vi "BATCH 4.vi"() -> ()   [LabVIEW 2019]
uses:
  <vilib>/LabVIEW Interface for Arduino/Type Defs/Pin Mode.ctl
  <vilib>/LabVIEW Interface for Arduino/LabVIEW Interface for Arduino.lvlib
  <vilib>/ptbypt/NI_PtbyPt.lvlib
panel:
  out "Boolean 7":bool
  out "Boolean 6":bool
  out "Boolean 5":bool
  out "Boolean 4":bool
  out "Boolean 2":bool
  out "Boolean":bool
  in  "stop":bool
  out "String":string="Device under standby/Monitoring Mode"
  out "O2 Valve ON/OFF Status":bool
  out "Respiration Graph":dynamicdata(graph)
  out "Sensor Output Voltage":dbl(knob) scale=0.0..5.0
  # "O2 INHALE LIMITER"
  # "TEAM MEMBERS' NAMES:\n\nJANANISHREE V (191BM119)\nKAVINKUMAR V S (191BM121)\nKAVIYASRI S (191BM122)\nKISHORE S (191BM123)\nNAVYA C PRAKASH (191BM128)"
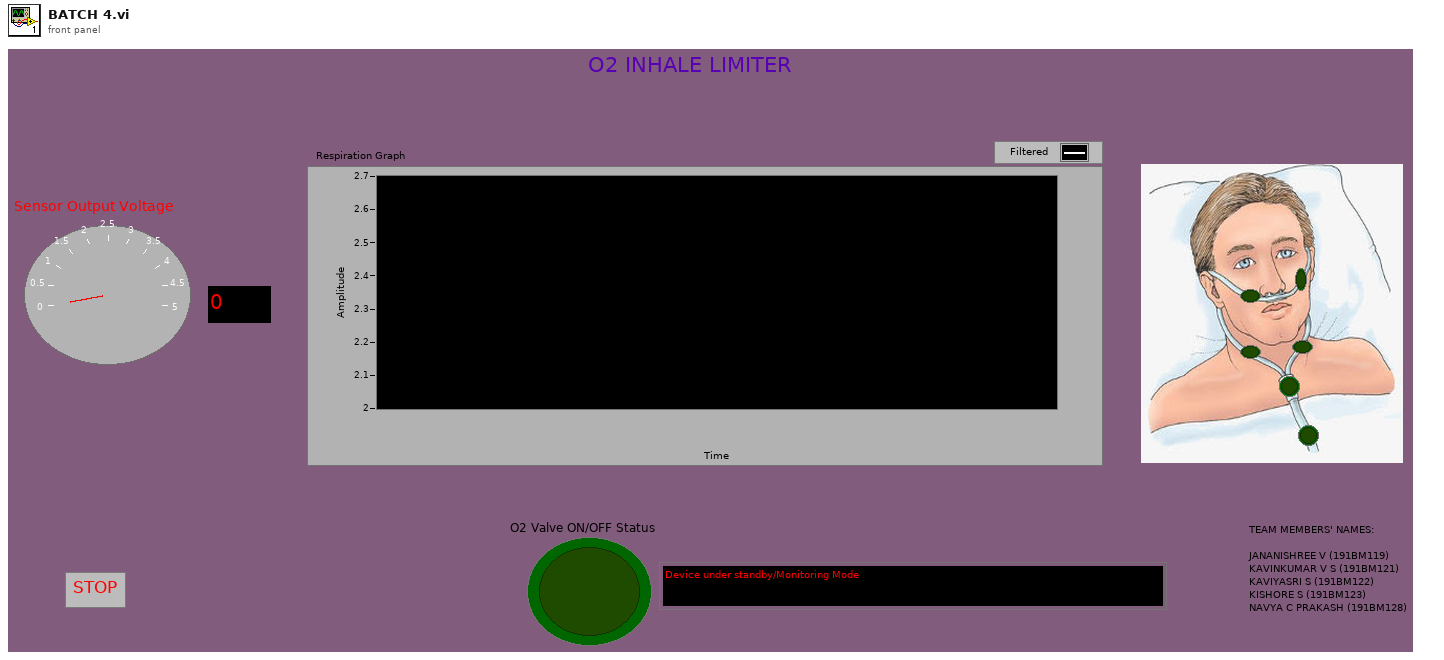
[diagram p1: front panel]
types:
  T1 = typedef "LabVIEW Interface for Arduino.lvlib/Arduino Resource.ctl" = cluster{"VISA resource":refnum<visa-resource-name>, "Board Type":T2, "Connection Type":enum8{"USB / Serial"}, "Bytes Per Packet (15)":u8}
  T2 = typedef "LabVIEW Interface for Arduino.lvlib/Board Type.ctl" = enum16{"Uno", "Dimuelanove w/Atmega 328", "Mega 2560"}
  T3 = typedef "LabVIEW Interface for Arduino.lvlib/Pin Mode.ctl" = enum8{"Input", "Output"}
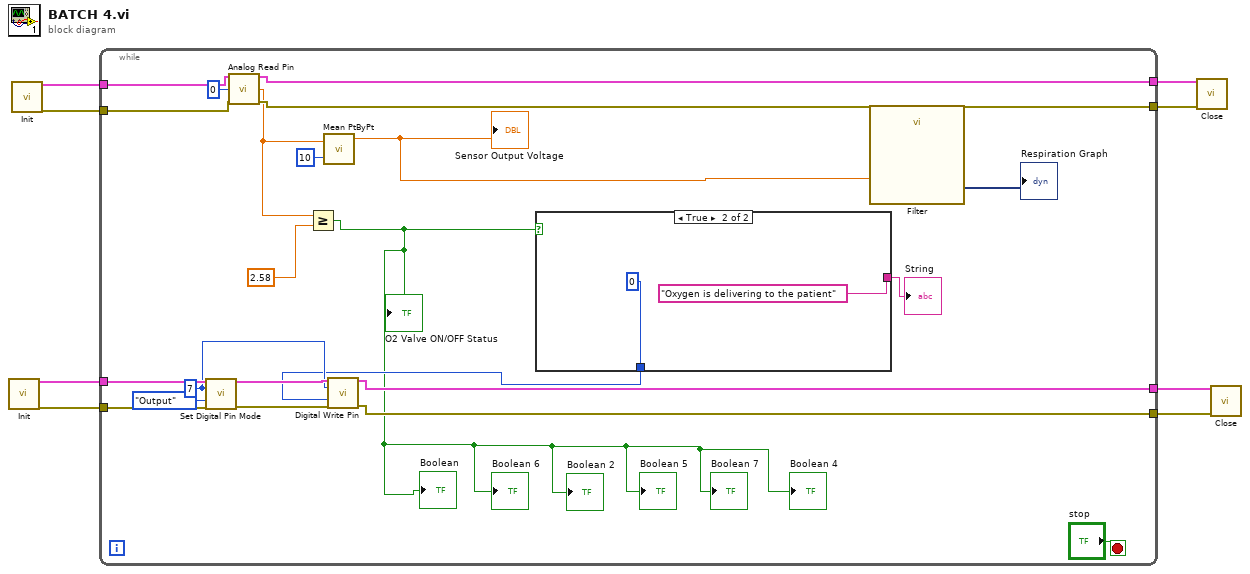
[diagram p0: block diagram]
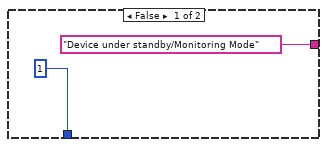
[diagram p2: hidden frame]
diagram:
  n1 = call <vilib>:"Init.vi"() -> ("Arduino Resource"=w4:T1, "error out"=w2:errorcluster)  [unwired: 18 in]
  n2 = call <vilib>:"Init.vi"() -> ("Arduino Resource"=w8:T1, "error out"=w6:errorcluster)  [unwired: 18 in]
  n3 = while {
    tunnel: w8 -> [w29]
    tunnel: [w28] -> w7
    tunnel: w6 -> [w27]
    tunnel: [w26] -> w5
    tunnel: w4 -> [w24]
    tunnel: [w22] -> w3
    tunnel: w2 -> [w21]
    tunnel: [w19] -> w1
    stop <- "stop" stop-if-true
    w17 = u8 7 ("Digital I/O Pin")
    n4 = call <vilib>:"Set Digital Pin Mode.vi"("Arduino Resource"=w24, "Digital I/O Pin"=w17, "Pin Mode (Input)"=Pin_Mode."Output", "error in"=w21) -> ("Arduino Resource"=w23:T1, "error out"=w20:errorcluster)  [unwired: 10 in]
    n5 = call <vilib>:"Analog Read Pin.vi"("Arduino Resource"=w29, "Analog Input Pin (0)"=u8 0, "error in"=w27) -> ("Arduino Resource"=w28:T1, "Voltage"=w12:dbl, "error out"=w26:errorcluster)  [unwired: 10 in]
    n6 = Greater Or Equal?(x=w12, y=2.58) -> (x >= y?=w9:bool)
    "O2 Valve ON/OFF Status" <- w9
    "Boolean" <- w9
    "Boolean 6" <- w9
    "Boolean 2" <- w9
    "Boolean 5" <- w9
    "Boolean 7" <- w9
    "Boolean 4" <- w9
    n7 = call <vilib>:"Mean PtByPt.vi"("x"=w12, "sample length"=10) -> ("mean"=w14:dbl)  [unwired: 2 in, 1 out]
    "Sensor Output Voltage" <- w14
    n8 = case shown="True" w9 {
      tunnel: [1 0] -> w15
      tunnel: ["Device under standby/Monitoring Mode" "Oxygen is delivering to the patient"] -> w10
      frame False {
      }
      frame True {
      }
    }
    "String" <- w10
    n9 = call <vilib>:"Digital Write Pin.vi"("Arduino Resource"=w23, "Digital I/O Pin (0)"=w17, "Value (0)"=w15, "error in"=w20) -> ("Arduino Resource"=w22:T1, "error out"=w19:errorcluster)  [unwired: 10 in]
    n10 = call "Filter"("Signal"=w14) -> ("Filtered Signal"=→"Respiration Graph":dynamicdata)  [unwired: 9 in, 1 out]
  }
  n11 = call <vilib>:"Close.vi"("Arduino Resource"=w7, "error in"=w5) -> ()  [unwired: 13 in, 1 out]
  n12 = call <vilib>:"Close.vi"("Arduino Resource"=w3, "error in"=w1) -> ()  [unwired: 13 in, 1 out]
